vi "Create and Open TDMS File.vi"(6 "Samples Per Channel":i32, 8 "Error In":errorcluster, 9 "TDMS Group Name":string, 10 "TDMS Channel Name":string[](array[string]), 11 "TDMS File Path":path) -> (0 "Error Out":errorcluster, 3 "TDMS File Ref Out":refnum<k34>)   [LabVIEW 2014]
doc: "Create a Single TDMS File with the inputted parameters and padd the file with a default value (i.e 0.001). Return the reference to this file."
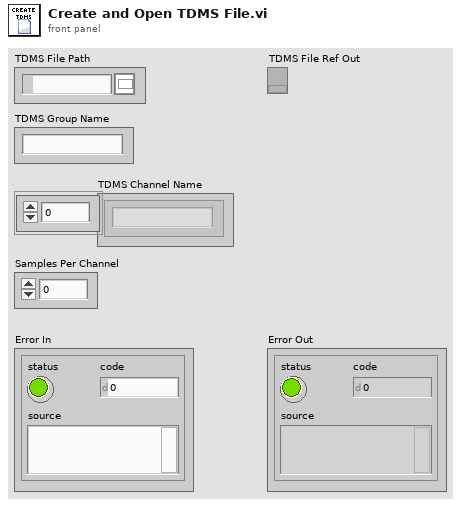
[diagram p1: front panel]
types:
  T1 = enum16{"open", "open or create", "create or replace", "create", "open (read-only)"}
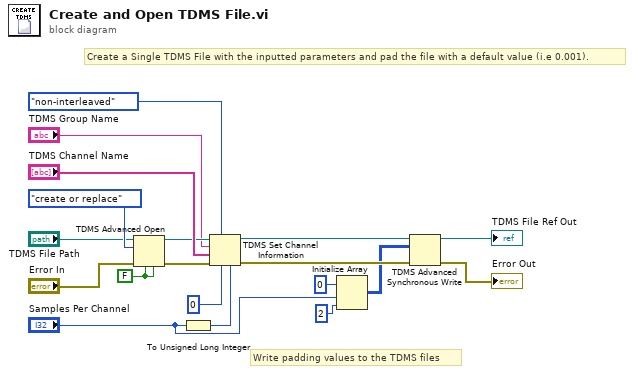
[diagram p0: block diagram]
diagram:
  w1 = FALSE ("enable asynchronous? (T)")
  # "Create a Single TDMS File with the inputted parameters and pad the file with a default value (i.e 0.001)."
  # "Write padding values to the TDMS files"
  n1 = TDMS Advanced Open(4:w1, 6:w1, 8:"Error In", 10:T1."create or replace" ("File Operation"), 11:"TDMS File Path") -> (0:w10:errorcluster, 3:w9:refnum<k34>)  [unwired: 1 out]
  n2 = To Unsigned Long Integer(number="Samples Per Channel") -> (unsigned 32bit integer=w16:u32)
  n3 = TDMS Set Channel Information(4:w16, 6:i16 0 ("element"), 7:enum16{"non-interleaved", "interleaved"}."non-interleaved" ("data layout (0:non-interleaved)"), 8:w10, 9:"TDMS Channel Name", 10:"TDMS Group Name", 11:w9) -> (0:w13:errorcluster, 3:w12:refnum<k34>)
  n4 = Initialize Array(i16 0 ("element"), "Samples Per Channel", 2 ("dimension size")) -> (w3:i16[][])
  n5 = TDMS Advanced Synchronous Write(8:w13, 10:w3, 11:w12) -> (0:→"Error Out":errorcluster, 3:→"TDMS File Ref Out":refnum<k34>)
